vi "GUI_Bella_IP2.vi"() -> ()   [LabVIEW 2020]
uses:
  GUI_BELLA_ESP/Control 1.ctl
  Device Drivers/FilterWheels/posTypDef.ctl
  Shared/GUI_Template/GUI_master/tcp new data cluster.ctl
  <vilib>/vision/Image Controls.llb/IMAQ Image.ctl
panel:
  out "error IO 3":errorcluster
  in  "Position.Axis 2::23":dbl caption="Up/Down" min=-100000.0 max=100000.0 format="%.3g"
  in  "Position.Axis 3::23":dbl caption="Transverse" min=-100000.0 max=100000.0 format="%.3g"
  in  "Position.Axis 4::23":dbl caption="In/Out" min=-100000.0 max=100000.0 format="%.3g"
  in  "GUIdevice 24":string="IP2-Pico-WaterJet"
  in  "GUIdevice 23":string="IP2-Pico-catcher"
  in  "GUIdevice 22":string="IP2-MCD-NewmarkZ"
  in  "GUIdevice 21":string="IP2-MCD-NewmarkX"
  in  "GUIdevice 20":string="IP2-MCD-NewmarkY"
  in  "GUIdevice 18":string="IP2-FW-DiagTable"
  in  "Tab Control":enum32{"Motors", "Cameras"}(tab)
  in  "position::22":dbl caption="Scintillator" min=-50.0 max=320.0 format="%.3g"
  in  "Position.Axis 1::13":dbl caption="Camera" min=0.0 max=300.0 format="%.3g"
  in  "Position.Axis 3::24":dbl caption="tip/tilt z" min=-100000.0 max=100000.0 format="%.3g"
  in  "Position.Axis 4::24":dbl caption="tip/tilt x" min=-100000.0 max=100000.0 format="%.3g"
  in  "Position.Axis 2::24":dbl caption="rotation" min=-100000.0 max=100000.0 format="%.3g"
  in  "Position.Axis 1::24":dbl caption="tip/tilt y" min=-100000.0 max=100000.0 format="%.3g"
  in  "pos.Channel5::18":T1=enum."4" caption="M2 cam"
  in  "pos.Channel0::18":T1=enum."4" caption="ip2 HASO"
  in  "stop":bool
  in  "Position.Axis 3::3":T2 caption="IP2 M3 hrz" min=-20.0 max=20.0 format="%.3f"
  in  "Position.Axis 1::3":dbl caption="IP2 M6 hrz" min=-20.0 max=20.0 format="%.3g"
  in  "Position.Axis 3::4":dbl caption="IP2 M3 vrt" min=-20.0 max=20.0 format="%.3g"
  in  "Position.Axis 1::4":dbl=1.0 caption="IP2 M6 vrt (broken)" min=-100.0 max=100.0 format="%.3g"
  in  "Position.Axis 1::14":dbl=-1.68 caption="Focus Diag x" min=0.0 max=25.0 format="%.3g"
  in  "pos.Channel0::9":T1=enum."4" caption="MI FW"
  in  "position::21":dbl=-17.84 caption="Focus diag Z" min=-100.0 max=100.0 format="%.3g"
  in  "Position.Axis 2::14":T2 caption="x pos" min=-200.0 max=150.0 format="%.3f"
  in  "position::20":T2 caption="y pos" min=-25.0 max=20.0 format="%.3f"
  in  "Position.Axis 3::14":T2 caption="z pos" min=0.0 max=100.0 format="%.3f"
  in  "Position.Axis 3::15":string caption="Focus Diag y"
  out "IP2-CAM-2":T3(plugin-control)
  in  "TargetSize.Y::6":dbl=50.0 caption="Size Y" min=2.0 max=3000.0
  in  "Color 6":u32(colorbox)=16711680 caption="Color"
  in  "TargetSize.X::6":dbl=50.0 caption="Size X" min=2.0 max=3000.0
  in  "Target.Y::6":dbl=330.0 caption="Y" min=0.0 max=2000.0
  in  "Target.X::6":dbl=1320.0 caption="X" min=0.0 max=2000.0
  in  "exposure::6":dbl=0.07 caption="exposure" min=3.8e-05 max=1.0 format="%.3p"
  in  "exposure::7":dbl=0.015 caption="exposure" min=3.8e-05 max=1.0 format="%.3p"
  out "IP2-targetobs":T3(plugin-control)
  in  "TargetSize.Y::7":dbl=50.0 caption="Size Y" min=2.0 max=3000.0
  in  "Color 7":u32(colorbox)=16711680 caption="Color"
  in  "TargetSize.X::7":dbl=50.0 caption="Size X" min=2.0 max=3000.0
  in  "Target.Y::7":dbl=433.0 caption="Y" min=0.0 max=2000.0
  in  "Target.X::7":dbl=820.0 caption="X" min=0.0 max=2000.0
  in  "trigger::6":bool caption="Trigger"
  in  "trigger::7":bool caption="Trigger"
  out "image::7":T3(plugin-control) caption="M1 Cam"
  out "image::6":T3(plugin-control) caption="M1 Cam"
  in  "Position.Axis 1::17":dbl caption="TargetX" min=-200.0 max=200.0 format="%.3g"
  in  "Position.Axis 2::17":dbl caption="Peptide Stage" min=-200.0 max=150.0 format="%.3g"
  in  "Position.Axis 3::17":dbl caption="TargetZ" min=-100.0 max=50.0 format="%.3g"
  in  "GUIdevice 16":string="IP2-TC-ESP5"
  in  "GUIdevice 15":string="IP2-TC-ESP6"
  in  "Position.Axis 1::15":dbl caption="OPEN" min=0.0 max=2.9 format="%.3g"
  in  "GUIdevice 14":string="IP2-TC-ESP3"
  in  "Position.Axis 1::14":dbl caption="TapeDrive Z" min=0.0 max=25.0 format="%.3g"
  in  "Position.Axis 3::14":dbl=25.0 caption="Target scatter lens" min=0.0 max=100.0 format="%.3g"
  in  "GUIdevice 13":string="IP2-TC-ESP4"
  in  "Position.Axis 1::13":dbl caption="OAPT-Horz (Yaw)" min=0.0 max=300.0 format="%.3g"
  in  "Position.Axis 2::13":dbl caption="OAPT-Vert (Pitch)" min=-3.0 max=3.0 format="%.3g"
  in  "Position.Axis 3::13":dbl caption="Profiler Block" min=0.0 max=100.0 format="%.3g"
  in  "Position.Axis 1::12":dbl caption="IP2 M5 vrt" min=-100.0 max=100.0 format="%.3g"
  in  "Position.Axis 2::12":dbl caption="IP2 M6 (SFL) vrt" min=-150.0 max=150.0 format="%.3g"
  in  "Position.Axis 3::12":dbl caption="IP2 M3 (LFL) vrt" min=-20.0 max=20.0 format="%.3g"
  in  "Position.Axis 3::11":dbl caption="IP2 M3 (LFL) hrz" min=-20.0 max=20.0 format="%.3g"
  in  "Position.Axis 2::11":dbl caption="IP2 M6 (SFL) hrz" min=0.0 max=20.0 format="%.3g"
  in  "Position.Axis 1::11":dbl caption="IP2 M5 hrz" min=-20.0 max=20.0 format="%.3g"
  in  "GUIdevice 9":string="IP2-MI-FW"
  in  "GUIdevice 8":string="IP2-focusdiag-zy" caption="GUIdevice 4"
  in  "GUIdevice 7":string="IP2-targetobs"
  in  "GUIdevice 6":string="IP2-CAM-2" caption="GUIdevice 4"
  in  "GUIdevice 4":string="IP2-BTL-ESP2"
  in  "GUIdevice 3":string="IP2-BTL-ESP1"
  # "\"Focal Spot Horiz\""
  # "\"1in mirror (zaber)\""
  # "TC-ESP3"
  # "TC-ESP4"
  # "TC-ESP5"
  # "TC-ESP6"
  # "Target-XYZ"
  # "BTL-ESP1"
  # "BTL-ESP2"
  # "Waterjet picos"
  # "Waterjet Stages"
  # "Catcher picos"
  # "IN:         16.32+\nOUT:      67.42"
  # "IN:         36.7-\nOUT:      N/A"
  # "Proton spatial 1"
  # "IN:         73.69-\nOUT:       24"
  # "IN:         93.5\nOUT:       5"
  # "IN:         5\nOUT:      145"
  # "Microscope FS Mode IM"
  # "IN:         1.64\nOUT:       N/A"
  # "IN:         -16.17\nOUT:       N/A"
  # "IN:         141.76+\nOUT:       15"
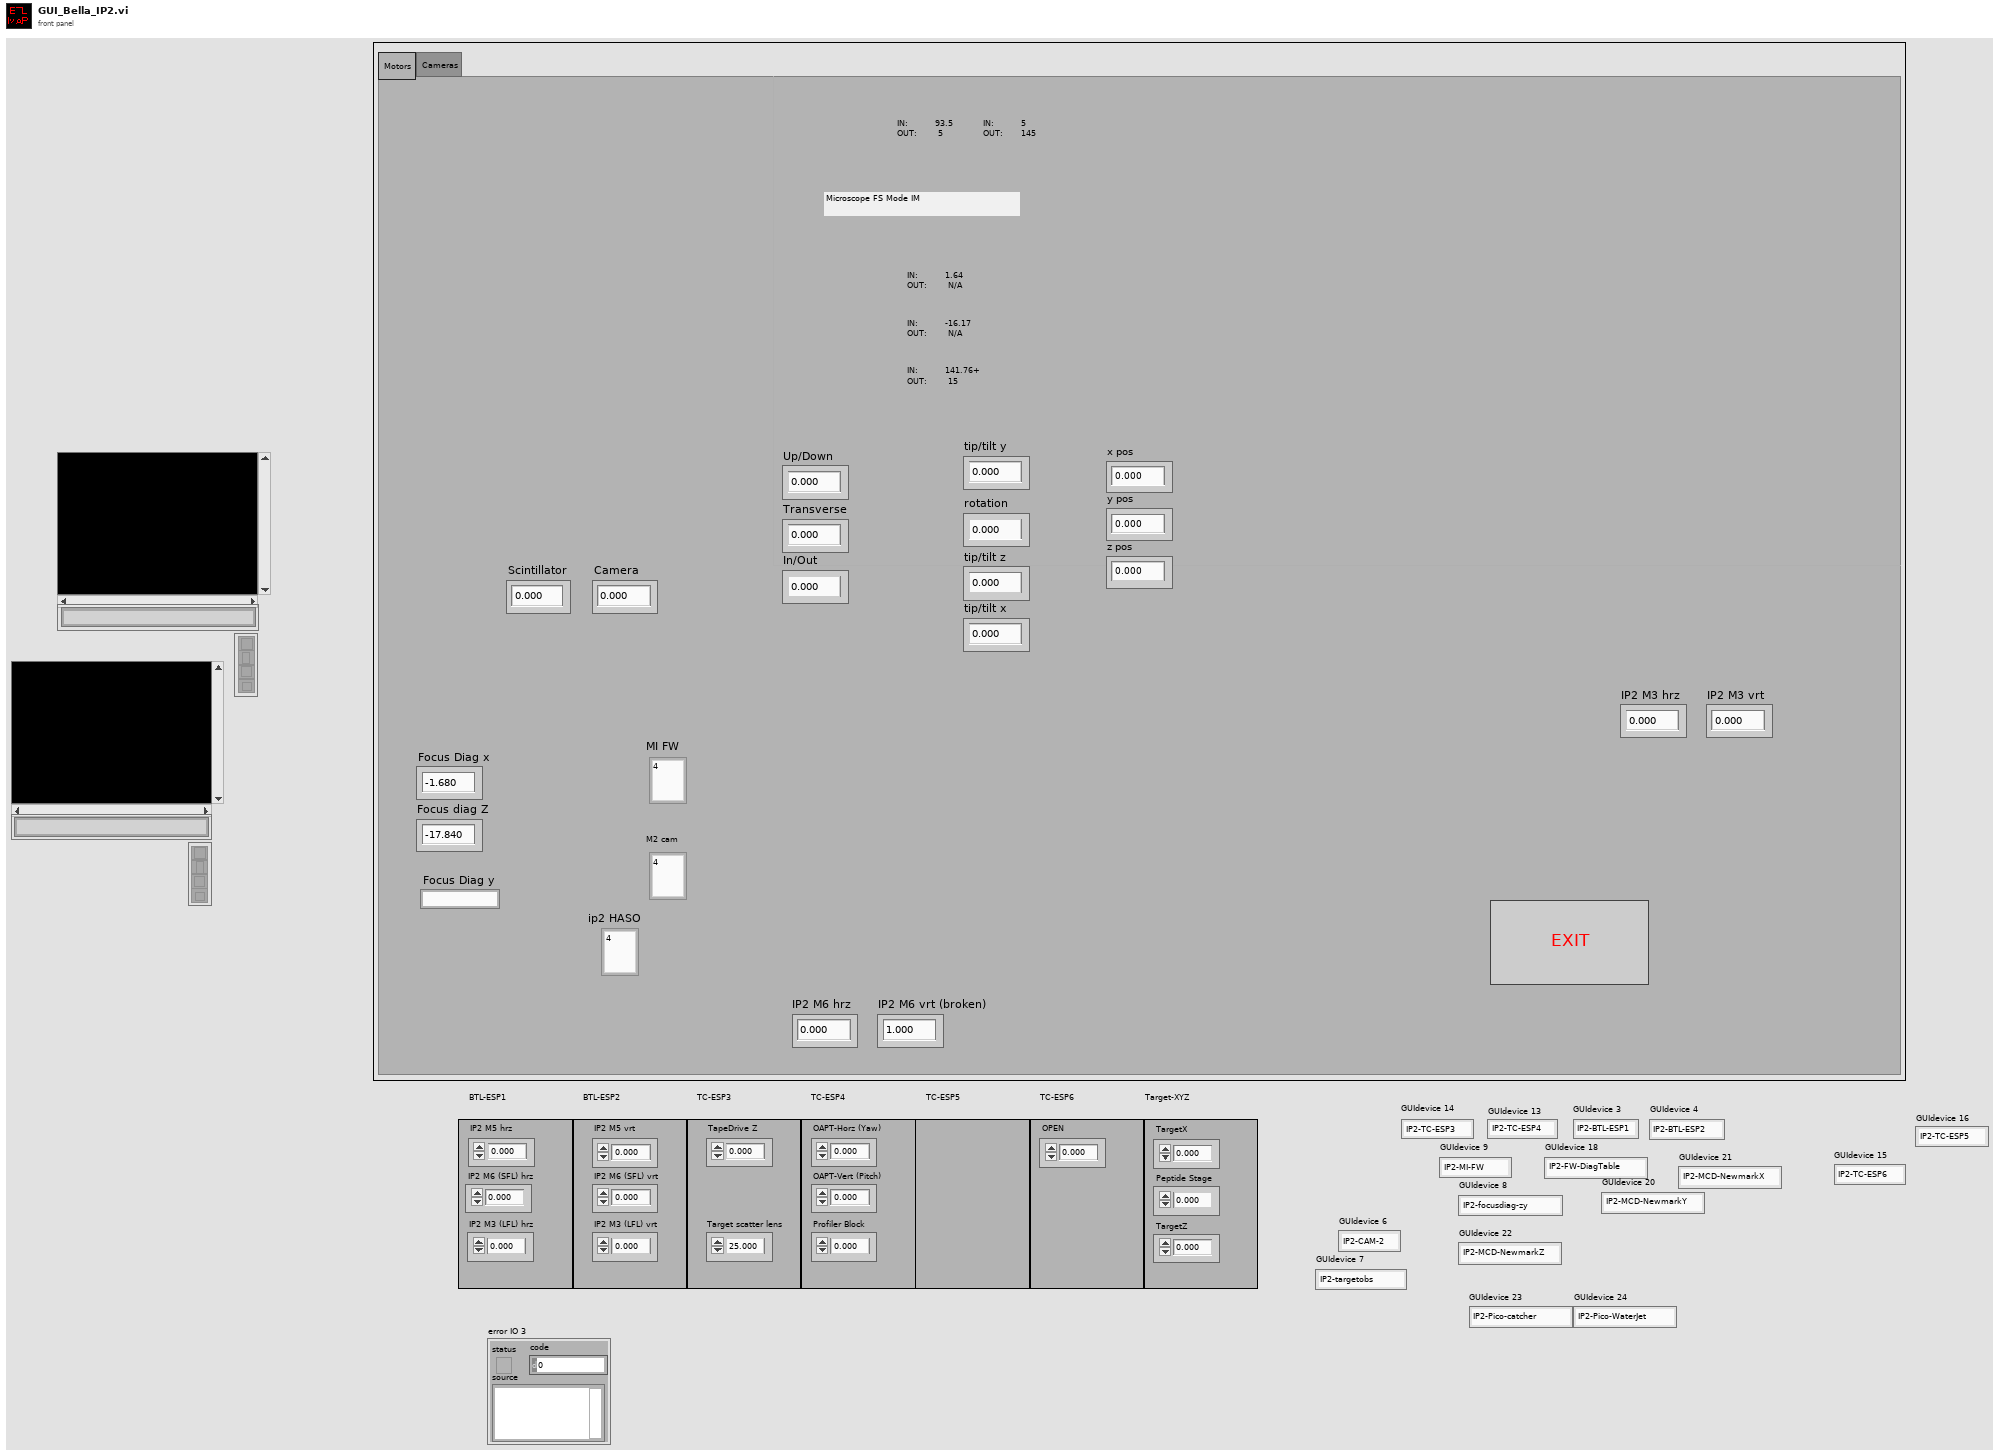
[diagram p1: front panel]
types:
  T1 = typedef "posTypDef.ctl" = enum16{"1", "2", "3", "4", "5", "6"}
  T2 = typedef "Control 1.ctl" = dbl
  T3 = typedef "IMAQ Image.ctl" = refnum<image>
  T4 = cluster{"Last update Cam1":u32, "Last update Cam2":u32, "Last update Cam3":u32, "Last update Cam4":u32, "Last update Cam5":u32, "Last update Cam6":u32, "Last update Cam7":u32, "Last update Cam8":u32}
  T5 = typedef "Image Type" = u32
  T6 = typedef "tcp new data cluster.ctl" = cluster{"EventEnum":enum16{"new data", "connection status update"}, "Device name":string}
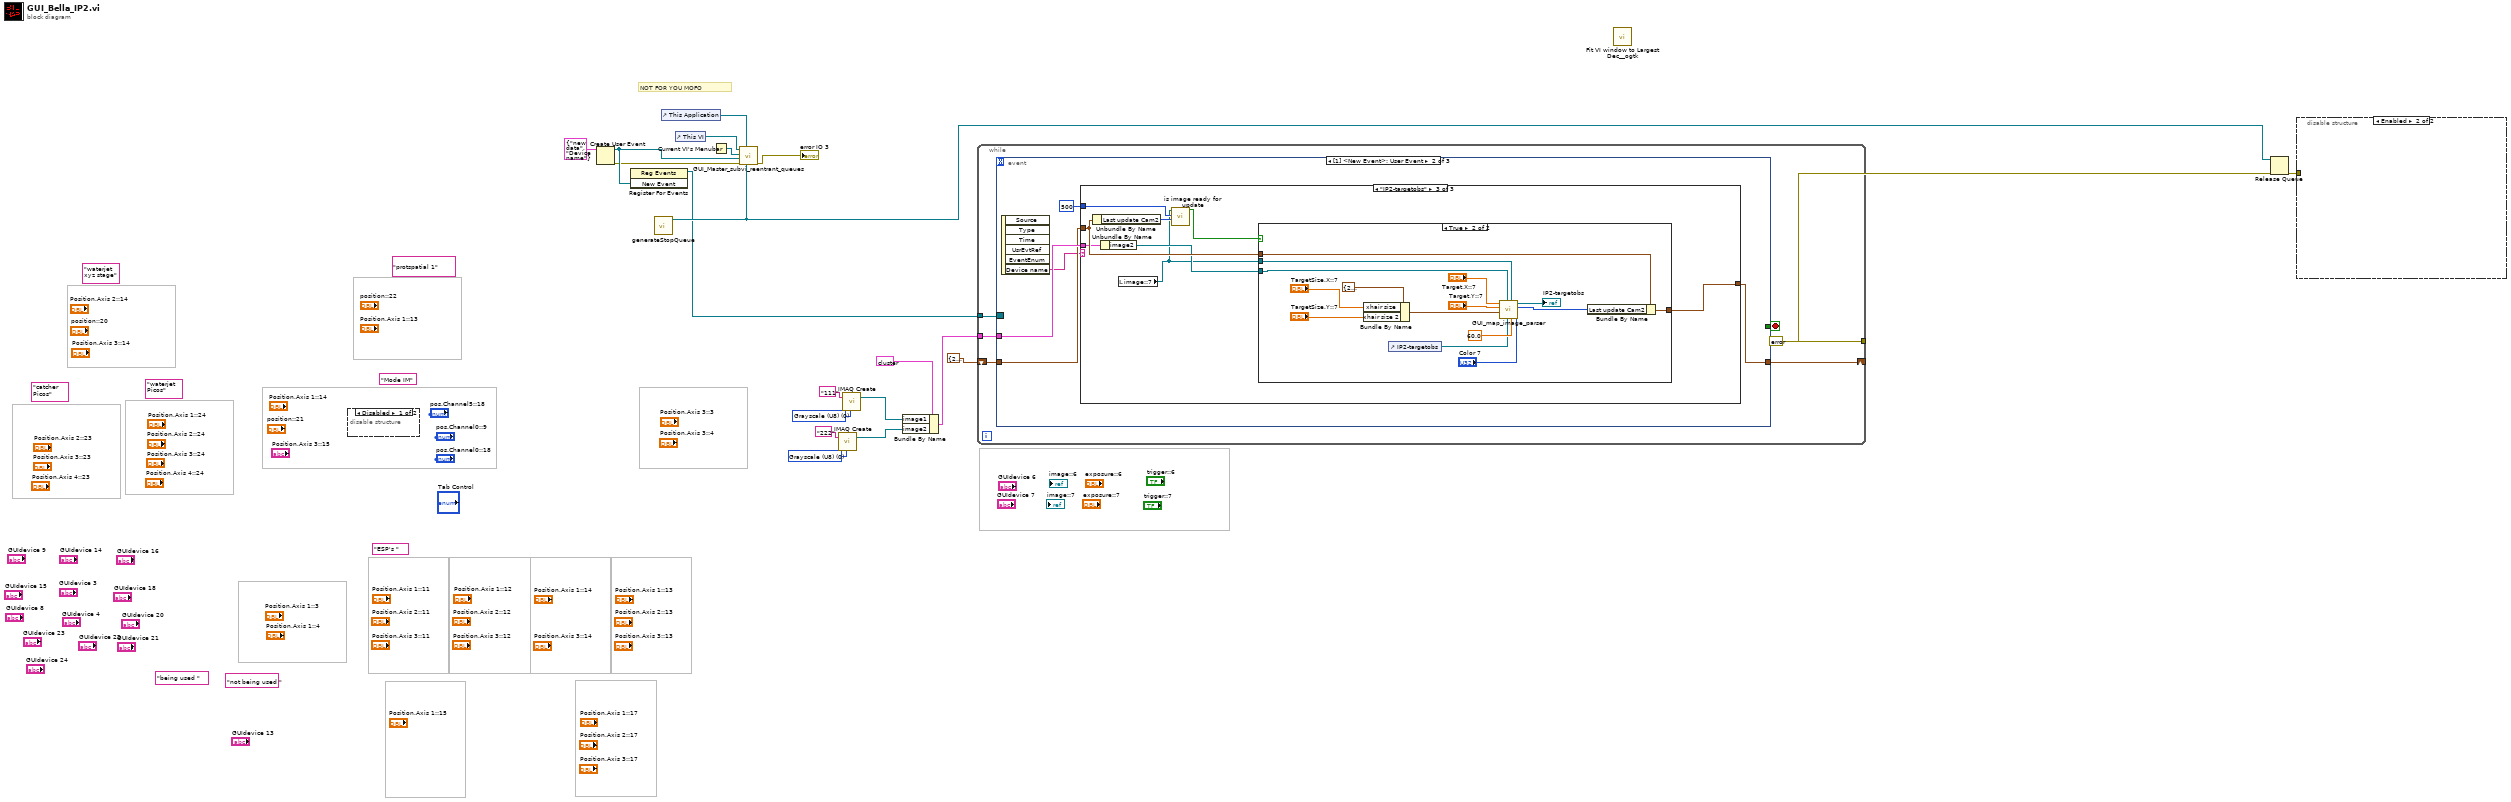
[diagram p0: block diagram]
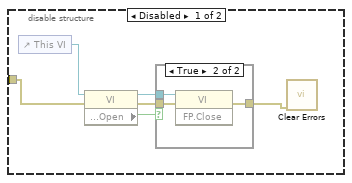
[diagram p3: hidden frame]
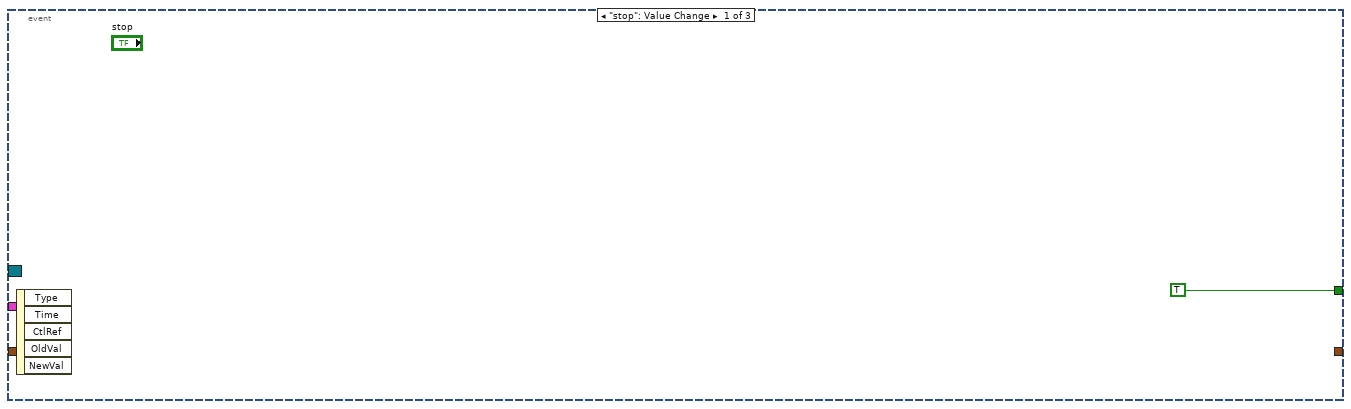
[diagram p5: hidden frame]
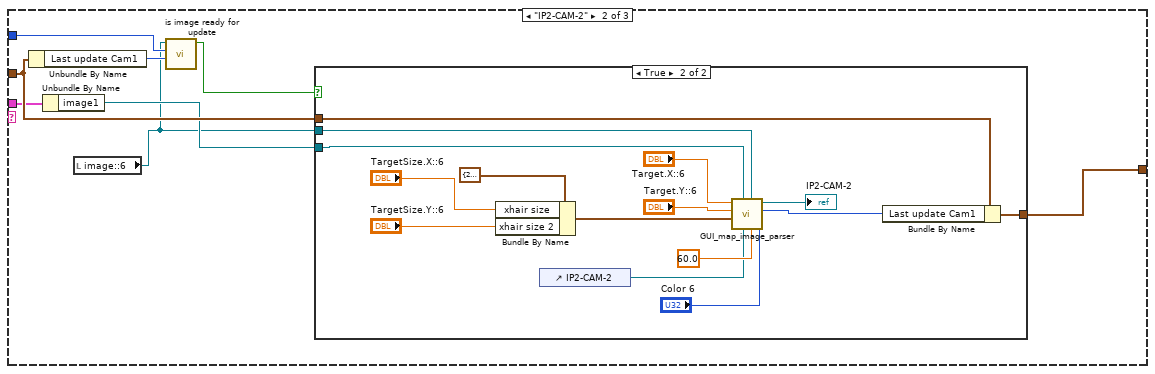
[diagram p7: hidden frame]
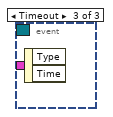
[diagram p10: hidden frame]
diagram:
  (unwired) "catcher Picos"
  (unwired) "waterjet Picos"
  (unwired) "protspatial 1"
  (unwired) "Mode IM"
  (unwired) "waterjet xyz stage"
  w8 = T5 0 items=["Grayscale (U8)", "Grayscale (I16)", "Grayscale (SGL)", "Complex (CSG)", "RGB (U32)", "HSL (U32)", "RGB (U64)", "Grayscale (U16)"] ("Image Type")
  w10 = T5 0 items=["Grayscale (U8)", "Grayscale (I16)", "Grayscale (SGL)", "Complex (CSG)", "RGB (U32)", "HSL (U32)", "RGB (U64)", "Grayscale (U16)"] ("Image Type")
  (unwired) "not being used "
  (unwired) "being used "
  (unwired) "ESP's "
  # "NOT FOR YOU MOFO"
  n1 = disable-structure shown="Disabled" {
    frame Disabled {
    }
    frame Enabled {
    }
  }
  n2 = Create User Event(user event datatype=T6 {"EventEnum"=enum."new data", "Device name"="Device name"} ("New Event")) -> (user event=w19:refnum<user-event>, error out=w18:errorcluster)  [unwired: 1 in]
  n3 = register-events(w19) -> (reference out=w11:refnum<event-registration>)  [unwired: 2 in, 1 out]
  n4 = call "generateStopQueue.vi"() -> ("STOP Queue out"=w14:refnum<queue>)  [unwired: 10 in, 1 out]
  n5 = control-ref of="This Application"() -> (w20:refnum<vi>)
  n6 = control-ref of="This VI"() -> (w15:refnum<vi>)
  n7 = Current VI's Menubar() -> (w16:refnum<k9>)
  n8 = call "GUI_Master_subvi_reentrant_queues.vi"("STOP Queue in"=w14, "This Application"=w20, "error in (no error)"=w18, "tcp data event"=w19, "Caller menu reference"=w16, "Caller VI ref"=w15) -> ("error out"=→"error IO 3":errorcluster)  [unwired: 5 in]
  n9 = call "IMAQ Create"("Image Name"="222", "Image Type"=w10) -> ("New Image"=w5:T3)  [unwired: 3 in, 1 out]
  n10 = call "IMAQ Create"("Image Name"="111", "Image Type"=w8) -> ("New Image"=w6:T3)  [unwired: 3 in, 1 out]
  n11 = Bundle By Name(cluster=cluster{"image1":T3, "image2":T3} {"image1"="image1", "image2"="image2"} ("input cluster"), "image1"=w6, "image2"=w5) -> (w3:cluster{"image1":T3, "image2":T3})
  n12 = while {
    tunnel: [errorcluster {"status"=FALSE, "code"=0, "source"=""} ("error in (no error)")] -> w13
    tunnel: w11 -> [w24]
    tunnel: w3 -> [w23]
    shift-right: [w21] -> _
    shift-left: T4 {"Last update Cam1"=200, "Last update Cam2"=200, "Last update Cam3"=200, "Last update Cam4"=200, "Last update Cam5"=200, "Last update Cam6"=200, "Last update Cam7"=200, "Last update Cam8"=200} -> [w22]
    stop <- w26 stop-if-true
    n13 = event shown="[1] <New Event>: User Event" {
      selector: w24 -> [_ _ _]
      dyn-events: _ -> [_ _ _]
      timeout: _ -> [_ _ _]
      tunnel: [TRUE ("stop") _ _] -> w26
      tunnel: w23 -> [_ w31 _]
      tunnel: w22 -> [_ w30 _]
      tunnel: [_ w28 _] -> w21
      event "stop": Value Change {
        n14 = event-data() -> ()  [unwired: 1 in, 5 out]
      }
      event User Event {
        n15 = event-data() -> ("Device name"=w29:string)  [unwired: 1 in, 5 out]
        n16 = case shown="\"IP2-targetobs\"" w29 {
          tunnel: w31 -> [_ w37 w61]
          tunnel: w30 -> [w33 w39 w63]
          tunnel: [w33 w38 w62] -> w28
          tunnel: u32 500 ("x-y") -> [_ w35 w59]
          frame "False", Default {
          }
          frame "IP2-CAM-2" {
            n17 = Unbundle By Name(w39) -> ("Last update Cam1"=w40:u32)
            n18 = Unbundle By Name(w37) -> ("image1"=w36:T3)
            n19 = local read "image::6"() -> (w34:T3)
            n20 = call "is image ready for update.vi"("Last update"=w40, "min time between updates"=w35, "image ref in"=w34) -> ("update image"=w41:bool)  [unwired: 8 in]
            n21 = case shown="True" w41 {
              tunnel: w39 -> [w42 w57]
              tunnel: [w42 w56] -> w38
              tunnel: w34 -> [_ w55]
              tunnel: w36 -> [_ w47]
              frame False {
              }
              frame True {
                n22 = Bundle By Name(cluster=cluster{"xhair size":dbl, "xhair size 2":dbl} {"xhair size"=20.0, "xhair size 2"=20.0} ("size"), "xhair size"="TargetSize.X::6", "xhair size 2"="TargetSize.Y::6") -> (w48:cluster{"xhair size":dbl, "xhair size 2":dbl})
                n23 = control-ref of="IP2-CAM-2"() -> (w43:refnum<vi>)
                n24 = call "GUI_map_image_parser.vi"("color"="Color 6", "zoom#"=60.0, "Image Src"=w55, "Ctl Refnum"=w43, "Image Dst"=w47, "size"=w48, "target y"="Target.Y::6", "target x"="Target.X::6") -> ("ms timer out"=w52:u32, "Img out"=→"IP2-CAM-2":T3)  [unwired: 2 in]
                n25 = Bundle By Name(cluster=w57, "Last update Cam1"=w52) -> (w56:T4)
              }
            }
          }
          frame "IP2-targetobs" {
            n26 = Unbundle By Name(w63) -> ("Last update Cam2"=w64:u32)
            n27 = Unbundle By Name(w61) -> ("image2"=w60:T3)
            n28 = local read "image::7"() -> (w58:T3)
            n29 = call "is image ready for update.vi"("Last update"=w64, "min time between updates"=w59, "image ref in"=w58) -> ("update image"=w65:bool)  [unwired: 8 in]
            n30 = case shown="True" w65 {
              tunnel: w63 -> [w66 w81]
              tunnel: [w66 w80] -> w62
              tunnel: w58 -> [_ w79]
              tunnel: w60 -> [_ w71]
              frame False {
              }
              frame True {
                n31 = Bundle By Name(cluster=cluster{"xhair size":dbl, "xhair size 2":dbl} {"xhair size"=20.0, "xhair size 2"=20.0} ("size"), "xhair size"="TargetSize.X::7", "xhair size 2"="TargetSize.Y::7") -> (w72:cluster{"xhair size":dbl, "xhair size 2":dbl})
                n32 = control-ref of="IP2-targetobs"() -> (w67:refnum<vi>)
                n33 = call "GUI_map_image_parser.vi"("color"="Color 7", "zoom#"=60.0, "Image Src"=w79, "Ctl Refnum"=w67, "Image Dst"=w71, "size"=w72, "target y"="Target.Y::7", "target x"="Target.X::7") -> ("ms timer out"=w76:u32, "Img out"=→"IP2-targetobs":T3)  [unwired: 2 in]
                n34 = Bundle By Name(cluster=w81, "Last update Cam2"=w76) -> (w80:T4)
              }
            }
          }
        }
      }
      event Timeout {
        n35 = event-data() -> ()  [unwired: 1 in, 2 out]
      }
    }
  }
  n36 = call <userlib>:"Fit VI window to Largest Dec__ogtk.vi"() -> ()  [unwired: 6 in, 2 out]
  n37 = Release Queue(queue=w14, error in (no error)=w13) -> (error out=w12:errorcluster)  [unwired: 1 in, 2 out]
  n38 = disable-structure shown="Enabled" {
    disable-tunnel: w12 -> [w83 _]
    frame Disabled {
      n39 = control-ref of="This VI"() -> (w84:refnum<vi>)
      n40 = property class="VI"(reference=w84, error in=w83) -> (reference out=w86:refnum<vi>, error out=w87:errorcluster, "Front Panel.Open"=w85:bool)
      n41 = case shown="True" w85 {
        tunnel: [w88 w91] -> w82
        tunnel: w87 -> [w88 w90]
        tunnel: w86 -> [_ w89]
        frame False {
        }
        frame True {
          n42 = invoke class="VI" method="FP.Close"(reference=w89, error in=w90) -> (error out=w91:errorcluster)  [unwired: 1 in, 2 out]
        }
      }
      n43 = call <vilib>:"Clear Errors.vi"("error in (no error)"=w82) -> ()  [unwired: 5 in, 2 out]
    }
    frame Enabled {
    }
  }
